vi "Wingbeat Amplitude Extraction (FPGA main).vi"() -> ()   [LabVIEW 2013, in "FPGA Image Processing.lvlib"]
uses:
  FPGA Image Processing.lvlib
  LabVIEW/Vision/Vision-RIO/Vision-RIO/Common/CL Configuration.ctl
  LabVIEW/Vision/Vision-RIO/Vision-RIO/Common/CL Signal Mapping.ctl
  <vilib>/Platform/TimedLoop/XDataNode/timing_clust.ctl
  <vilib>/Platform/TimedLoop/XDataNode/nitl_modes.ctl
  <vilib>/Platform/TimedLoop/XDataNode/wakeup.ctl
  <vilib>/rvi/Emulation/niFpgaSctlEmulationGetInTimedLoop.vi
  <vilib>/rvi/Emulation/niFpgaEmulationReportErrorSimple.vi
  <vilib>/rvi/eio/common/nirviEmuTemplateMethod_errors.vi
  <vilib>/rvi/Emulation/niFpgaGetClockAttributes.vi
  <vilib>/rvi/Emulation/niFpgaCriticalErrorInLSC.vi
  LabVIEW/Vision/Vision-RIO/Vision-RIO/Common/CL Data to Pixels/10 Tap 8-Bit.vi
  <vilib>/rvi/Emulation/niFpgaProcessEmulError.vi
  <vilib>/Platform/TimedLoop/XDataNode/XDataNode.xnode
  <vilib>/eio/EIONode/EIONode.xnode
  <vilib>/Platform/TimedLoop/XDataNode/XDNodeRunTimeDep.lvlib
panel:
  out "Right Wing Sector Mean Pixel Values":fxp<+/-,32,16>[](array[numeric])
  out "Left Wing Sector Mean Pixel Values":fxp<+/-,32,16>[](array[numeric])
  out "Right Wing Sector Pixel Count":u16[](array[numeric])
  out "Left Wing Sector Pixel Count":u16[](array[numeric])
  in  "Pixel":T1
  in  "Wing ROIs":T2
  out "Right Wing Sector Pixel Values":u16[](array[numeric])
  out "Left Wing Sector Pixel Values":u16[](array[numeric])
  in  "NumWingSectors":u8
  in  "UART.Transmit":bool
  in  "UART.Tx Data":u8[](array[numeric])=[0, 0, 0, 0, 0, 0, 0, 0, 0, 0] format="%02x"
  in  "UART.Set Baud Rate":bool
  in  "UART.Byte Mode":bool=TRUE
  out "UART.Rx Ready":bool
  out "UART.Break Indicator":bool
  out "UART.Framing Error":bool
  out "UART.Overrun Error":bool
  out "UART.Tx Ready":bool
  out "UART.Rx Data":u8 format="%02x"
  in  "UART.Receive":bool
  in  "UART.Baud Rate":u8
  in  "Acq Control.Ignore DVAL":bool
  in  "Acq Control.Cancel Acq":bool
  in  "Acq Control.Acquire":bool
  out "Acq Status.Frames Acq'd":u32
  out "Acq Status.Lines Per Frame":u32
  out "Acq Status.Clocks Per Line":u32
  in  "Acq Control.Frames To Acq":u32
  out "Acq Status.Acq In Progress":bool
  in  "Acq Control.Line Scan Height":u32
  in  "Acq Control.Initialize":bool
  out "Acq Status.Initialized":bool
  in  "CL Config.DVAL Active High":bool=TRUE
  in  "CL Config.FVAL Active High":bool=TRUE
  in  "CL Config.LVAL Active High":bool=TRUE
  in  "CL Config.Spare Active High":bool=TRUE
  in  "CL Config.Line Scan":bool
  in  "CL Config.Signal Mapping":T3=enum."Basler 10-tap"
  in  "CL Config.Configuration":T4=enum."Full"
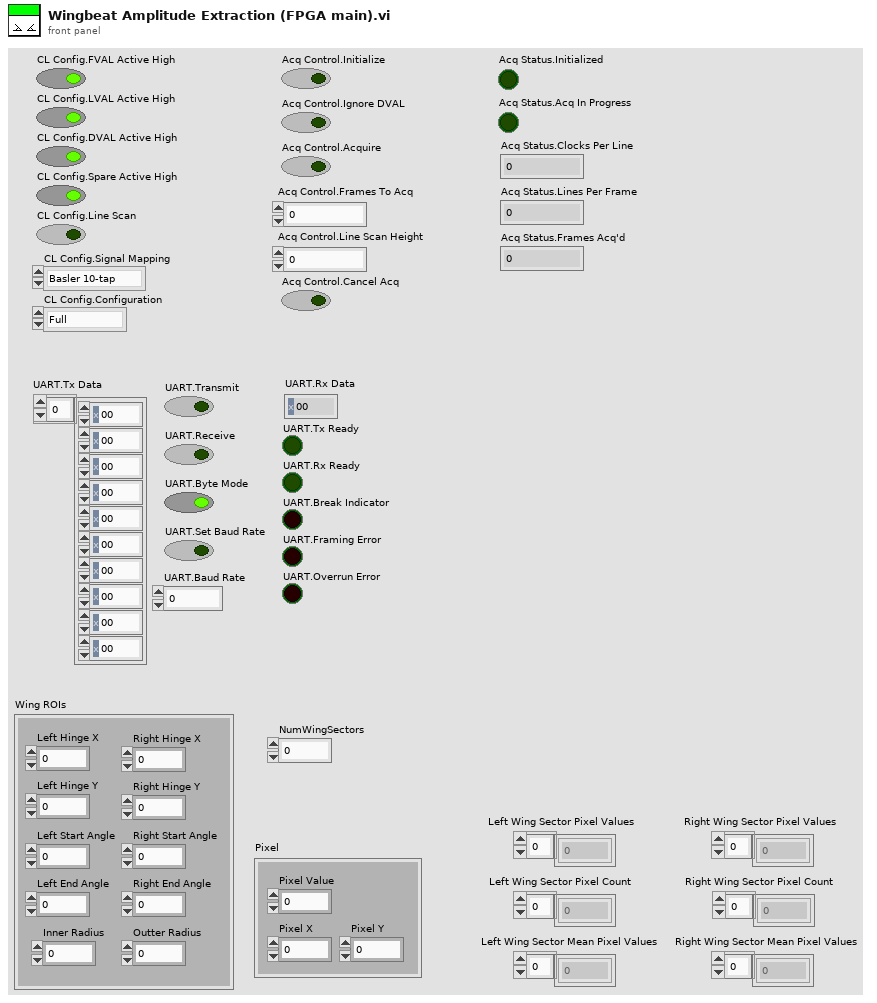
[diagram p1: front panel]
types:
  T1 = cluster{"Pixel Value":u8, "Pixel X":u16, "Pixel Y":u16}
  T2 = cluster{"Left Hinge X":u16, "Left Hinge Y":u16, "Inner Radius":u16, "Outter Radius":u16, "Right Hinge X":u16, "Right Hinge Y":u16, "Right Start Angle":i16, "Right End Angle":i16, "Left Start Angle":i16, "Left End Angle":i16}
  T3 = typedef "CL Signal Mapping.ctl" = enum8{"Standard", "Basler 10-tap", "Vosskühler 10-tap"}
  T4 = typedef "CL Configuration.ctl" = enum8{"Base", "Medium", "Full"}
  T5 = typedef "XDNodeRunTimeDep.lvlib/timing_clust.ctl" = cluster{"Expected End [f-1]":u64, "Actual End [f-1]":u64, "Finished Late? [f-1]":bool, "Expected End [i-1]":u64, "Actual End [i-1]":u64, "Finished Late? [i-1]":bool, "Expected Start [i]":u64, "Actual Start [i]":u64, "Expected Start [f]":u64, "Actual Start [f]":u64, "Source Name":string, "Structure Name":string, "Period":i64, "Deadline":i64, "Offset":i64, "Start":i64, "Priority":i32, "Timeout":i32, "Mode":T6, "Wakeup Reason":T7, "Error":errorcluster, "Source Type":string, "Secondary Source Type":string, "Global End Time":u64, "Global Start Time":u64, "Frame Duration":u64, "Iteration Duration":u64, "Assigned CPU":i32, "I/O Scan Engine Mode":u32}
  T6 = typedef "XDNodeRunTimeDep.lvlib/nitl_modes.ctl" = enum32{"No Change", "Process missed periods, maintain original phase", "Discard missed periods, maintain original phase", "Process missed periods, ignore original phase", "Discard missed periods, ignore original phase"}
  T7 = typedef "XDNodeRunTimeDep.lvlib/wakeup.ctl" = enum32{"Normal", "Aborted", "Asynchronous wakeup", "Timing source error", "Timed loop error", "Timeout"}
  T8 = cluster{"Enables Valid":bool, "Frame Valid":bool, "Line Valid":bool, "Data Valid":bool}
  T9 = cluster{"Pixel 0":u8, "Pixel 1":u8, "Pixel 2":u8, "Pixel 3":u8, "Pixel 4":u8, "Pixel 5":u8, "Pixel 6":u8, "Pixel 7":u8, "Pixel 8":u8, "Pixel 9":u8}
  T10 = cluster{"Tx Data":u8[], "Transmit":bool, "Receive":bool, "Byte Mode":bool, "Set Baud Rate":bool, "Baud Rate":u8}
  T11 = cluster{"Rx Data":u8, "Turn Off Transmit":bool, "Turn Off Receive":bool, "Turn Off Set Baud Rate":bool, "Tx Ready":bool, "Rx Ready":bool, "Break Indicator":bool, "Framing Error":bool, "Overrun Error":bool}
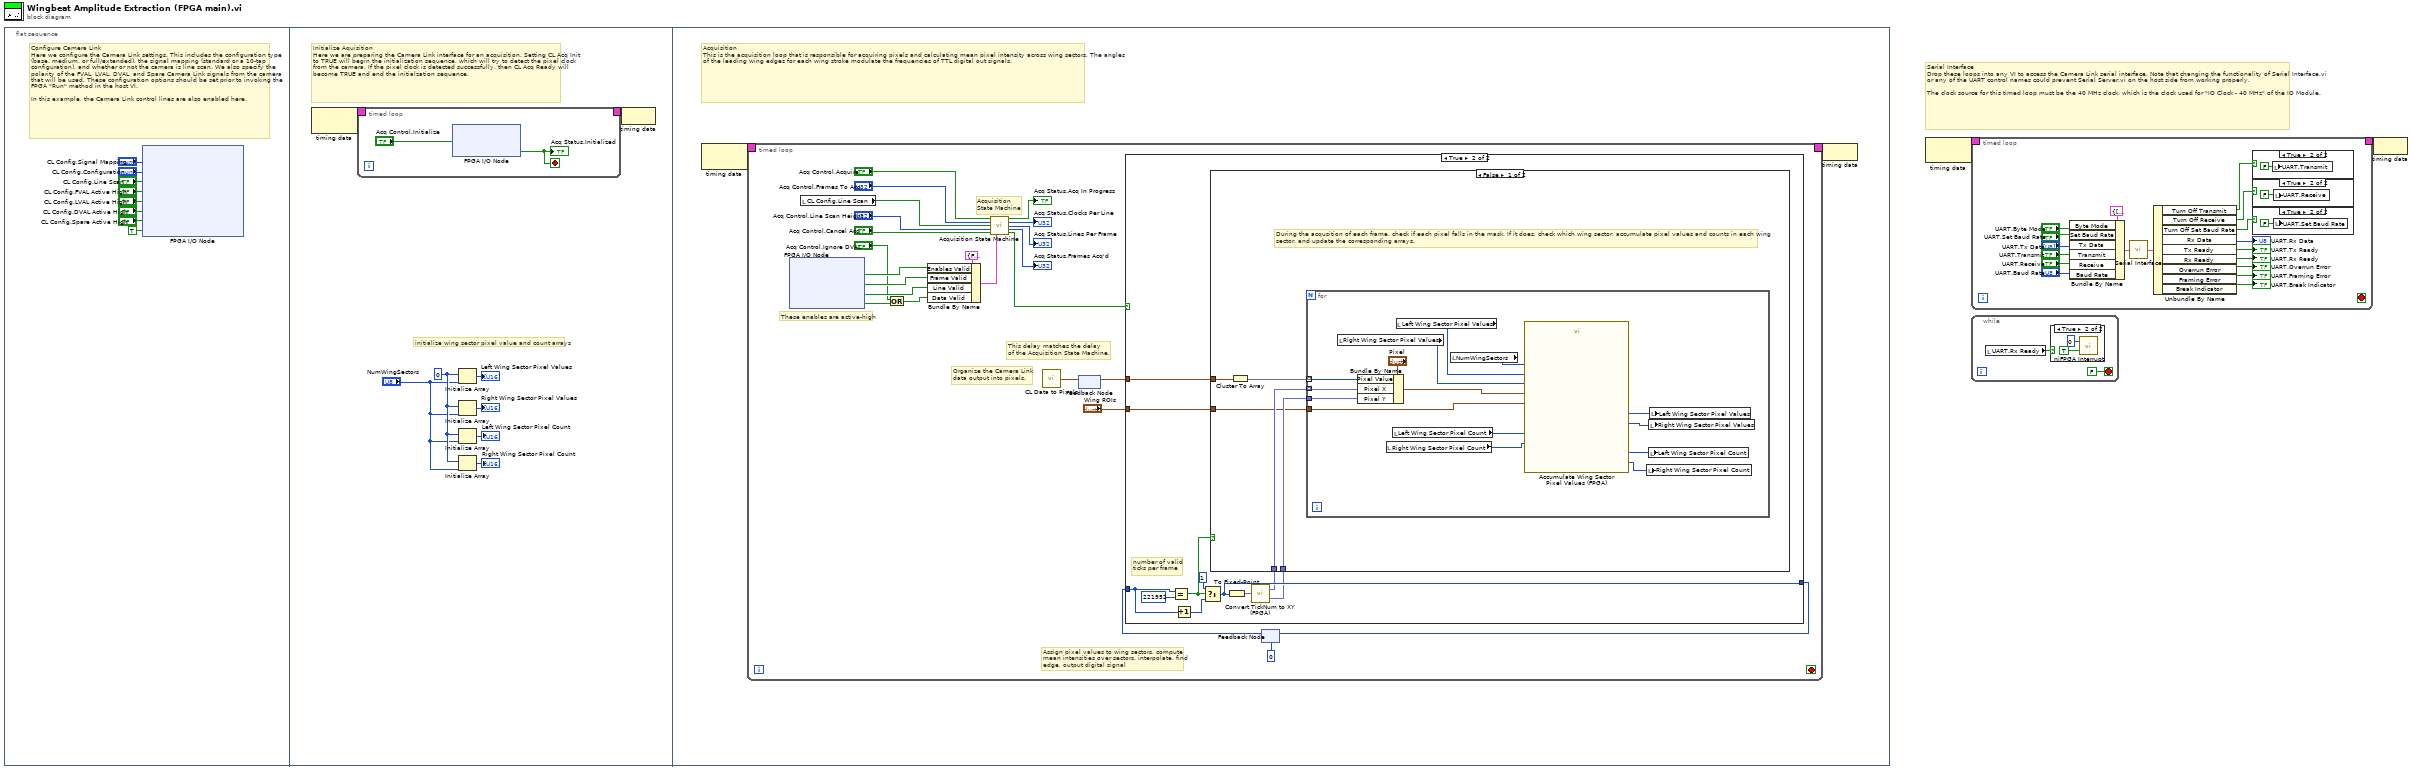
[diagram p0: block diagram]
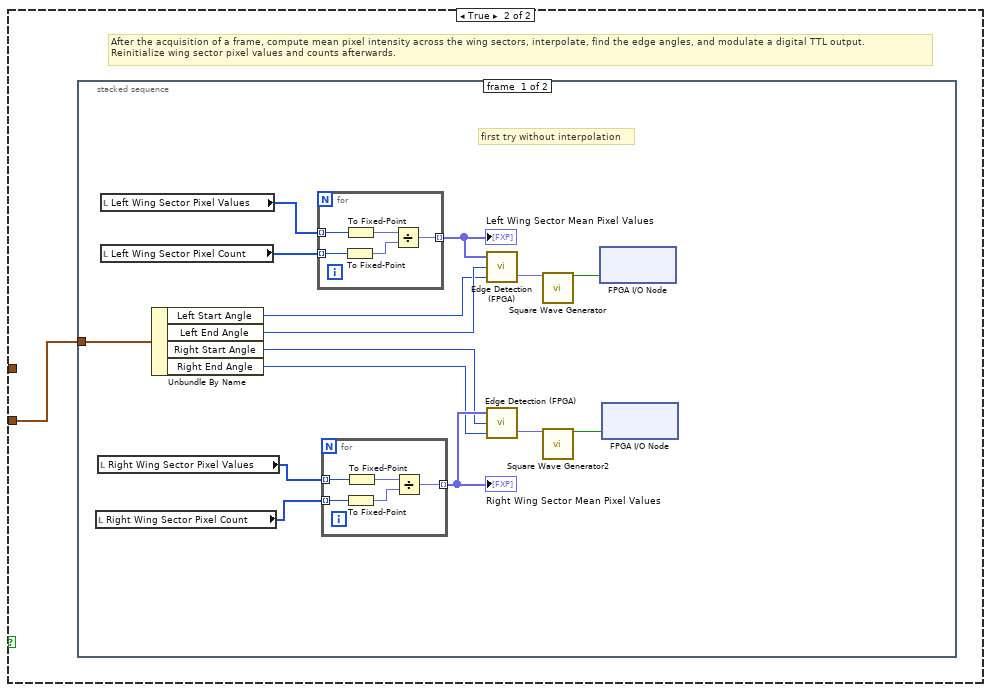
[diagram p7: hidden frame]
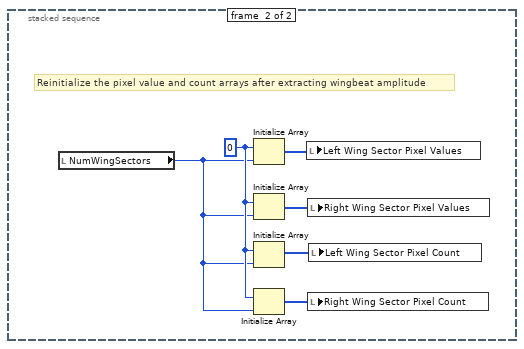
[diagram p8: hidden frame]
diagram:
  # "Serial Interface\nDrop these loops into any VI to access the Camera Link serial interface. Note that changing the functionality of Serial Interface.vi or any of the UART control names could prevent Serial Server.vi on the host side from working properly.\n\nThe clock source for this timed loop must be the 40 MHz clock, which is the clock used for \"IO Clock - 40 MHz\" of the IO Module."
  n1 = flat-sequence {
    frame #0 {
      # "Configure Camera Link\nHere we configure the Camera Link settings. This includes the configuration type (base, medium, or full/extended), the signal mapping (standard or a 10-tap configuration), and whether or not the camera is line scan. We also specify the polarity of the FVAL, LVAL, DVAL, and Spare Camera Link signals from the camera that will be used. These configuration options should be set prior to invoking the FPGA \"Run\" method in the host VI.\n\nIn this example, the Camera Link control lines are also enabled here."
      n2 = xnode "FPGA I/O Node"("CL Set Signal Mapping"="CL Config.Signal Mapping", "CL Set Configuration"="CL Config.Configuration", "CL Set Line Scan"="CL Config.Line Scan", "CL Set FVAL Active High"="CL Config.FVAL Active High", "CL Set LVAL Active High"="CL Config.LVAL Active High", "CL Set DVAL Active High"="CL Config.DVAL Active High", "CL Set Spare Active High"="CL Config.Spare Active High", "CL Control Enable"=TRUE ("IO Module\\CL Control Enable")) -> ()  [unwired: 8 in, 8 out]
    }
    frame #1 {
      w14 = u16 0 ("element")
      # "initialize wing sector pixel value and count arrays"
      # "Initialize Aquisition\nHere we are preparing the Camera Link interface for an acquisition. Setting CL Acq Init to TRUE will begin the initialization sequence, which will try to detect the pixel clock from the camera. If the pixel clock is detected successfully, then CL Acq Ready will become TRUE and end the initialzation sequence."
      n3 = node-c288() -> (w18:T5)  [unwired: 1 out]
      n4 = timed-loop {
        timing: w18 -> [_]
        timing-out: [_] -> w17
        stop <- w19 stop-if-true
        n5 = xnode "FPGA I/O Node"("CL Acq Init"="Acq Control.Initialize") -> ("CL Acq Ready"=w19:bool)  [unwired: 2 in, 2 out]
        "Acq Status.Initialized" <- w19
      }
      n6 = Initialize Array(w14, "NumWingSectors") -> (→"Left Wing Sector Pixel Values":u16[])
      n7 = Initialize Array(w14, "NumWingSectors") -> (→"Right Wing Sector Pixel Values":u16[])
      n8 = Initialize Array(w14, "NumWingSectors") -> (→"Left Wing Sector Pixel Count":u16[])
      n9 = Initialize Array(w14, "NumWingSectors") -> (→"Right Wing Sector Pixel Count":u16[])
      n10 = node-c288(w17) -> ()
    }
    frame #2 {
      # "Acquisition\nThis is the acquisition loop that is responsible for acquiring pixels and calculating mean pixel intensity across wing sectors. The angles of the leading wing edges for each wing stroke modulate the frequencies of TTL digital out signals."
      n11 = node-c288() -> (w26:T5)  [unwired: 1 in]
      n12 = timed-loop {
        timing: w26 -> [_]
        timing-out: [_] -> w25
        stop <- _ stop-if-true
        # "Assign pixel values to wing sectors, compute\nmean intensities over sectors, interpolate, find\nedge, output digital signal"
        # "Organize the Camera Link\ndata output into pixels."
        # "These enables are active-high"
        # "This delay matches the delay\nof the Acquisition State Machine."
        # "Acquisition\nState Machine"
        n13 = xnode "FPGA I/O Node"() -> ("CL Output Valid"=w42:bool, "CL Frame Valid"=w41:bool, "CL Line Valid"=w40:bool, "CL Data Valid"=w37:bool)  [unwired: 4 in, 4 out]
        n14 = local read "CL Config.Line Scan"() -> (w34:bool)
        n15 = Or(x="Acq Control.Ignore DVAL", y=w37) -> (x .or. y?=w36:bool)
        n16 = Bundle By Name(cluster=T8 {"Enables Valid"=FALSE, "Frame Valid"=FALSE, "Line Valid"=FALSE, "Data Valid"=FALSE} ("Enables"), "Enables Valid"=w42, "Frame Valid"=w41, "Line Valid"=w40, "Data Valid"=w36) -> (w39:T8)
        n17 = call "Acquisition State Machine.vi"("Acquire"="Acq Control.Acquire", "Frames to Acquire"="Acq Control.Frames To Acq", "Line Scan"=w34, "Line Scan Height"="Acq Control.Line Scan Height", "Cancel Acq"="Acq Control.Cancel Acq", "Enables"=w39) -> ("Acq In Progress"=→"Acq Status.Acq In Progress":bool, "Num Clocks Per Line"=→"Acq Status.Clocks Per Line":u32, "Num Lines Per Frame"=→"Acq Status.Lines Per Frame":u32, "Num Frames Acq'd"=→"Acq Status.Frames Acq'd":u32, "Capture Cycle"=w50:bool)  [unwired: 4 in, 1 out]
        n18 = call-poly "CL Data to Pixels.vi"() -> ("Pixels"=w29:T9)  [unwired: 1 in]
        n19 = feedback #1() -> (w28:T9)  [unwired: 1 in]
        n20 = feedback-in #1(w29) -> ()
        n21 = feedback #2(u32 0 ("y")) -> (w31:u32)
        n22 = case shown="True" w50 {
          tunnel: w31 -> [w51 w61]
          tunnel: [w51 w58] -> w32
          tunnel: w28 -> [_ w54]
          tunnel: "Wing ROIs" -> [_ w52]
          frame False {
          }
          frame True {
            # "number of valid\nticks per frame"
            n23 = Equal?(x=w61, y=u32 221952) -> (x = y?=w56:bool)
            n24 = Increment(x=w61) -> (x+1=w59:u32)
            n25 = Select(t=u32 1 ("y"), s=w56, f=w59) -> (s? t:f=w58:u32)
            n26 = To Fixed-Point(number=w58) -> (fixed-point=w57:fxp<+,32,32>)  [unwired: 1 in]
            n27 = call "Convert TickNum to XY (FPGA).vi"("numAcqTick"=w57) -> ("PixelXArray"=w55:fxp<+,1,1>[], "PixelY"=w53:fxp<+,12,12>)
            n28 = case shown="False" w56 {
              tunnel: w55 -> [w66 _]
              tunnel: w54 -> [w67 _]
              tunnel: w53 -> [w65 _]
              tunnel: w52 -> [w63 w83]
              frame False {
                # "During the acqusition of each frame, check if each pixel falls in the mask. If it does, check which wing sector, accumulate pixel values and counts in each wing\nsector, and update the corresponding arrays."
                n29 = Cluster To Array(cluster=w67) -> (array=w64:u8[])
                n30 = for {
                  tunnel: w66 -> [w80] mode=indexing
                  tunnel: w65 -> [w79]
                  tunnel: w64 -> [w78] mode=indexing
                  tunnel: w63 -> [w77]
                  n31 = local read "Right Wing Sector Pixel Values"() -> (w73:u16[])
                  n32 = Bundle By Name(cluster="Pixel", "Pixel Value"=w78, "Pixel X"=w80, "Pixel Y"=w79) -> (w81:T1)
                  n33 = local read "Right Wing Sector Pixel Count"() -> (w70:u16[])
                  n34 = local read "Left Wing Sector Pixel Count"() -> (w71:u16[])
                  n35 = local read "Left Wing Sector Pixel Values"() -> (w75:u16[])
                  n36 = local read "NumWingSectors"() -> (w76:u8)
                  n37 = call "Accumulate Wing Sector Pixel Values (FPGA).vi"("Right Wing Sector Pixel Count"=w70, "NumWingSectors"=w76, "Right Wing Sector Pixel Values"=w73, "Left Wing Sector Pixel Values"=w75, "Left Wing Sector Pixel Count"=w71, "Wing ROIs"=w77, "Pixel"=w81) -> ("Right Wing Sector Pixel Values 2"=w72:u16[], "Left Wing Sector Pixel Values 2"=w74:u16[], "Left Wing Sector Pixel Count 2"=w69:u16[], "Right Wing Sector Pixel Count 2"=w68:u16[])
                  n38 = local write "Right Wing Sector Pixel Count"(w68) -> ()
                  n39 = local write "Left Wing Sector Pixel Count"(w69) -> ()
                  n40 = local write "Right Wing Sector Pixel Values"(w72) -> ()
                  n41 = local write "Left Wing Sector Pixel Values"(w74) -> ()
                }
              }
              frame True {
                # "After the acquisition of a frame, compute mean pixel intensity across the wing sectors, interpolate, find the edge angles, and modulate a digital TTL output. \nReinitialize wing sector pixel values and counts afterwards."
                n42 = stacked-sequence {
                  tunnel: w83 -> [w94 _]
                  frame #0 {
                    # "first try without interpolation"
                    n43 = local read "Right Wing Sector Pixel Count"() -> (w95:u16[])
                    n44 = local read "Right Wing Sector Pixel Values"() -> (w96:u16[])
                    n45 = local read "Left Wing Sector Pixel Values"() -> (w98:u16[])
                    n46 = local read "Left Wing Sector Pixel Count"() -> (w97:u16[])
                    n47 = Unbundle By Name(w94) -> ("Left Start Angle"=w89:i16, "Left End Angle"=w90:i16, "Right Start Angle"=w86:i16, "Right End Angle"=w85:i16)
                    n48 = for {
                      tunnel: w98 -> [w108] mode=indexing
                      tunnel: w97 -> [w107] mode=indexing
                      tunnel: [w104] -> w91 mode=indexing
                      n49 = To Fixed-Point(number=w107) -> (fixed-point=w105:fxp<+,16,16>)  [unwired: 1 in]
                      n50 = To Fixed-Point(number=w108) -> (fixed-point=w106:fxp<+,16,16>)  [unwired: 1 in]
                      n51 = Divide(x=w106, y=w105) -> (x/y=w104:fxp<+,32,16>)
                    }
                    "Left Wing Sector Mean Pixel Values" <- w91
                    n52 = for {
                      tunnel: w96 -> [w99] mode=indexing
                      tunnel: w95 -> [w100] mode=indexing
                      tunnel: [w101] -> w87 mode=indexing
                      n53 = To Fixed-Point(number=w100) -> (fixed-point=w102:fxp<+,16,16>)  [unwired: 1 in]
                      n54 = To Fixed-Point(number=w99) -> (fixed-point=w103:fxp<+,16,16>)  [unwired: 1 in]
                      n55 = Divide(x=w103, y=w102) -> (x/y=w101:fxp<+,32,16>)
                    }
                    "Right Wing Sector Mean Pixel Values" <- w87
                    n56 = call "Edge Detection (FPGA).vi"("Mask End Angle"=w89, "Mask Start Angle"=w90, "Mean Pixel Values By Sector"=w91) -> ("Edge Angle"=w88:fxp<+/-,32,16>)  [unwired: 1 out]
                    n57 = call "Edge Detection (FPGA).vi"("Mask End Angle"=w85, "Mask Start Angle"=w86, "Mean Pixel Values By Sector"=w87) -> ("Edge Angle"=w84:fxp<+/-,32,16>)  [unwired: 1 out]
                    n58 = call "Square Wave Generator"("frequency (periods/tick)"=w88) -> ("square wave out"=w93:bool)  [unwired: 14 in]
                    n59 = call "Square Wave Generator2"("frequency (periods/tick)"=w84) -> ("square wave out"=w92:bool)  [unwired: 14 in]
                    n60 = xnode "FPGA I/O Node"("TTL 0"=w93) -> ()  [unwired: 1 in, 1 out]
                    n61 = xnode "FPGA I/O Node"("TTL 1"=w92) -> ()  [unwired: 1 in, 1 out]
                  }
                  frame #1 {
                    w114 = u16 0 ("element")
                    # "Reinitialize the pixel value and count arrays after extracting wingbeat amplitude"
                    n62 = local read "NumWingSectors"() -> (w113:u8)
                    n63 = Initialize Array(w114, w113) -> (w112:u16[])
                    n64 = Initialize Array(w114, w113) -> (w111:u16[])
                    n65 = Initialize Array(w114, w113) -> (w110:u16[])
                    n66 = Initialize Array(w114, w113) -> (w109:u16[])
                    n67 = local write "Left Wing Sector Pixel Values"(w112) -> ()
                    n68 = local write "Right Wing Sector Pixel Values"(w111) -> ()
                    n69 = local write "Right Wing Sector Pixel Count"(w109) -> ()
                    n70 = local write "Left Wing Sector Pixel Count"(w110) -> ()
                  }
                }
              }
            }
          }
        }
        n71 = feedback-in #2(w32) -> ()
      }
      n72 = node-c288(w25) -> ()
    }
  }
  n73 = node-c288() -> (w2:T5)  [unwired: 1 out]
  n74 = timed-loop {
    timing: w2 -> [_]
    timing-out: [_] -> w1
    stop <- _ stop-if-true
    n75 = Bundle By Name(cluster=T10 {"Tx Data"=[0, 0, 0, 0, 0, 0, 0, 0, 0, 0], "Transmit"=FALSE, "Receive"=FALSE, "Byte Mode"=TRUE, "Set Baud Rate"=FALSE, "Baud Rate"=0} ("UART Inputs"), "Byte Mode"="UART.Byte Mode", "Set Baud Rate"="UART.Set Baud Rate", "Tx Data"="UART.Tx Data", "Transmit"="UART.Transmit", "Receive"="UART.Receive", "Baud Rate"="UART.Baud Rate") -> (w119:T10)
    n76 = call "Serial Interface.vi"("UART Inputs"=w119) -> ("UART Outputs"=w131:T11)
    n77 = Unbundle By Name(w131) -> ("Turn Off Transmit"=w124:bool, "Turn Off Receive"=w125:bool, "Turn Off Set Baud Rate"=w121:bool, "Rx Data"=→"UART.Rx Data":u8, "Tx Ready"=→"UART.Tx Ready":bool, "Rx Ready"=→"UART.Rx Ready":bool, "Overrun Error"=→"UART.Overrun Error":bool, "Framing Error"=→"UART.Framing Error":bool, "Break Indicator"=→"UART.Break Indicator":bool)
    n78 = case shown="True" w124 {
      frame False {
      }
      frame True {
        n79 = local write "UART.Transmit"(FALSE ("UART.Transmit")) -> ()
      }
    }
    n80 = case shown="True" w125 {
      frame False {
      }
      frame True {
        n81 = local write "UART.Receive"(FALSE ("UART.Receive")) -> ()
      }
    }
    n82 = case shown="True" w121 {
      frame False {
      }
      frame True {
        n83 = local write "UART.Set Baud Rate"(FALSE ("UART.Receive")) -> ()
      }
    }
  }
  n84 = while {
    stop <- FALSE stop-if-true
    n85 = local read "UART.Rx Ready"() -> (w143:bool)
    n86 = case shown="True" w143 {
      frame False {
      }
      frame True {
        n87 = call <vilib>:"niFPGA Interrupt.vi"("Wait Until Cleared (F)"=TRUE ("Wait Until Cleared"), "IRQ Number (0)"=u8 0 ("IRQ Number")) -> ()  [unwired: 1 in]
      }
    }
  }
  n88 = node-c288(w1) -> ()
